vi "timer.vi"() -> ()   [LabVIEW 2023]
panel:
  out "Simulation time 2":dbl
  in  "stop":bool
  out "Simulation time":dbl
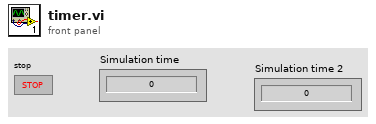
[diagram p1: front panel]
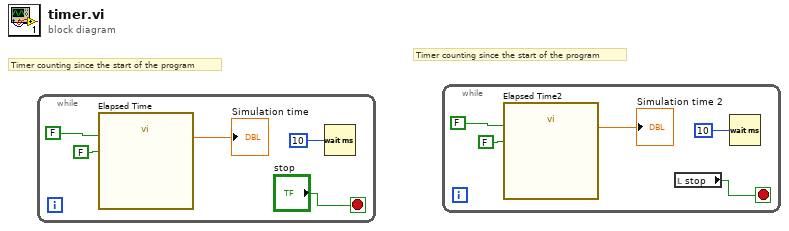
[diagram p0: block diagram]
diagram:
  # "Timer counting since the start of the program"
  # "Timer counting since the start of the program"
  n1 = while {
    stop <- "stop" stop-if-true
    n2 = call "Elapsed Time"("Reset"=FALSE, "Auto Reset"=FALSE) -> ("Elapsed Time (s)"=→"Simulation time":dbl)  [unwired: 10 in, 7 out]
    n3 = Wait (ms)(milliseconds to wait=u32 10) -> ()  [unwired: 1 out]
  }
  n4 = while {
    stop <- w6 stop-if-true
    n5 = call "Elapsed Time2"("Reset"=FALSE, "Auto Reset"=FALSE) -> ("Elapsed Time (s)"=→"Simulation time 2":dbl)  [unwired: 10 in, 7 out]
    n6 = local read "stop"() -> (w6:bool)
    n7 = Wait (ms)(milliseconds to wait=u32 10) -> ()  [unwired: 1 out]
  }
